vi "UTM_to_String.vi"(8 "error in":errorcluster, 11 "UTM Location":T1 {"North" format="%#_10f"; "East" format="%#_8f"}) -> (0 "error out":errorcluster, 3 "UTM String":string)   [LabVIEW 2011]
uses:
  2 Typedefs/UTM Location.ctl
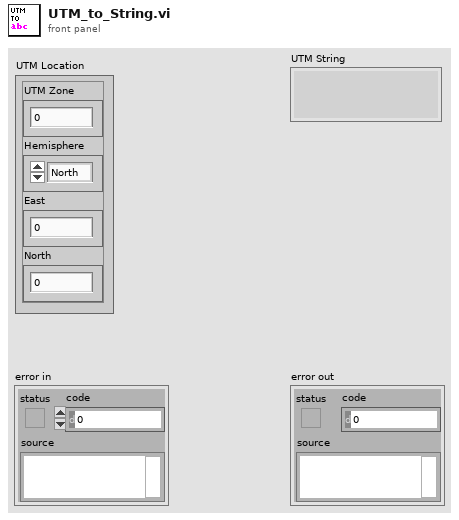
[diagram p1: front panel]
types:
  T1 = typedef "UTM Location.ctl" = cluster{"UTM Zone":dbl, "Hemisphere":enum16{"North", "South"}, "East":dbl, "North":dbl}
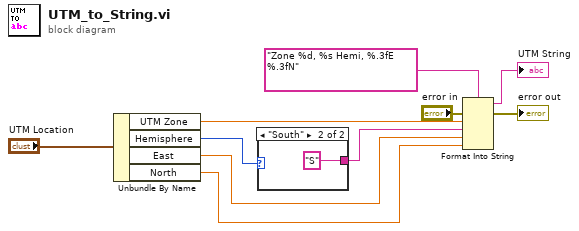
[diagram p0: block diagram]
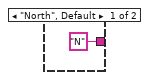
[diagram p2: hidden frame]
diagram:
  n1 = Unbundle By Name("UTM Location") -> ("UTM Zone"=w8:dbl, "Hemisphere"=w7:enum16{"North", "South"}, "East"=w5:dbl, "North"=w4:dbl)
  n2 = case shown="\"South\"" w7 {
    tunnel: ["N" ("input 2") "S" ("input 2")] -> w6
    frame "North", Default {
    }
    frame "South" {
    }
  }
  n3 = Format Into String(format string="Zone %d, %s Hemi, %.3fE %.3fN", error in="error in", w8, w6, w5, w4) -> (resulting string=→"UTM String":string, error out=→"error out":errorcluster)  [unwired: 1 in]
